vi "Temp_Calc.vi"(10 "TempCoeff":T1, 11 "raw_temp":u32) -> (1 "tfine":dbl, 2 "Temperature":dbl)   [LabVIEW 2020, in "BMP208.lvclass"]
uses:
  BMP208.lvclass
  Controls/td_cluster_Temp_Coeff.ctl
panel:
  out "tvar1":dbl format="%09.5f"
  out "tvar2":dbl
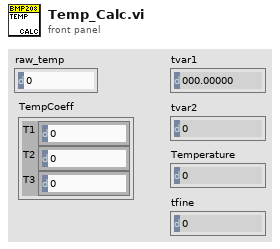
[diagram p1: front panel]
types:
  T1 = typedef "BMP208.lvclass/td_cluster_Temp_Coeff.ctl" = cluster{"T1":u16, "T2":i16, "T3":i16}
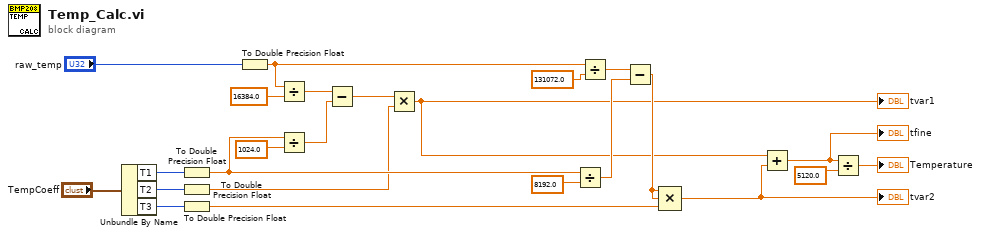
[diagram p0: block diagram]
diagram:
  n1 = Unbundle By Name("TempCoeff") -> ("T1"=w3:u16, "T2"=w2:i16, "T3"=w1:i16)
  n2 = To Double Precision Float(number=w3) -> (double precision float=w12:dbl)
  n3 = To Double Precision Float(number=w2) -> (double precision float=w11:dbl)
  n4 = To Double Precision Float(number=w1) -> (double precision float=w10:dbl)
  n5 = To Double Precision Float(number="raw_temp") -> (double precision float=w13:dbl)
  n6 = Divide(x=w13, y=16384.0) -> (x/y=w7:dbl)
  n7 = Divide(x=w12, y=1024.0) -> (x/y=w6:dbl)
  n8 = Subtract(x=w7, y=w6) -> (x-y=w9:dbl)
  n9 = Multiply(x=w9, y=w11) -> (x*y=w8:dbl)
  "tvar1" <- w8
  n10 = Divide(x=w12, y=8192.0) -> (x/y=w19:dbl)
  n11 = Divide(x=w13, y=131072.0) -> (x/y=w20:dbl)
  n12 = Subtract(x=w20, y=w19) -> (x-y=w18:dbl)
  n13 = Compound Arithmetic op=MULTIPLY(w18, w18, w10) -> (w5:dbl)
  "tvar2" <- w5
  n14 = Add(x=w8, y=w5) -> (x+y=w15:dbl)
  "tfine" <- w15
  n15 = Divide(x=w15, y=5120.0) -> (x/y=→"Temperature":dbl)
